vi "Timestamp from dat file.vi"(10 "dat file path":path) -> (2 "time stamp":timestamp)   [LabVIEW 2018]
uses:
  <vilib>/Utility/miscctls.llb/LVDateTimeRec.ctl
panel:
  in  "date time rec":T1
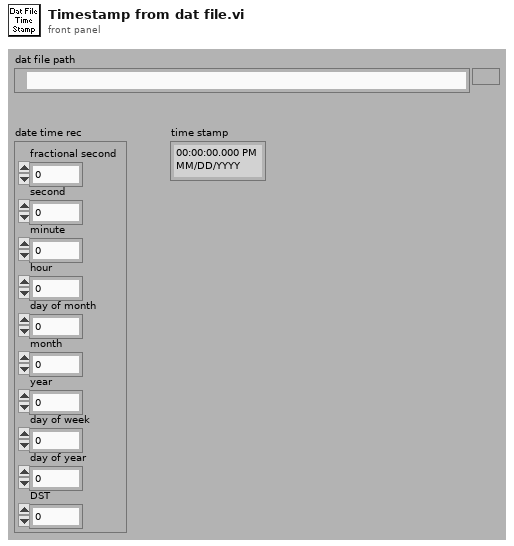
[diagram p1: front panel]
types:
  T1 = typedef "LVDateTimeRec.ctl" = cluster{"fractional second":dbl, "second":i32, "minute":i32, "hour":i32, "day of month":i32, "month":i32, "year":i32, "day of week":i32, "day of year":i32, "DST":i32}
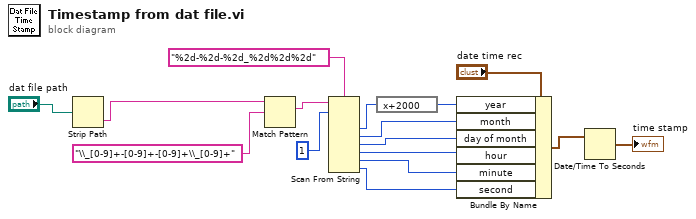
[diagram p0: block diagram]
diagram:
  n1 = Strip Path(path="dat file path") -> (name=w5:string)  [unwired: 1 out]
  n2 = Match Pattern(string=w5, regular expression="\\_[0-9]+-[0-9]+-[0-9]+\\_[0-9]+") -> (match substring=w2:string)  [unwired: 1 in, 3 out]
  n3 = Scan From String(format string="%2d-%2d-%2d_%2d%2d%2d", input string=w2, initial scan location=u32 1) -> (output 1=w15:i32, output 2=w13:i32, output 3=w12:i32, output 4=w11:i32, output 5=w10:i32, output 6=w9:i32)  [unwired: 7 in, 3 out]
  n4 = expression code="x+2000"(w15) -> (w14:i32)
  n5 = Bundle By Name(cluster="date time rec", "year"=w14, "month"=w13, "day of month"=w12, "hour"=w11, "minute"=w10, "second"=w9) -> (w8:T1)
  n6 = Date/Time To Seconds(2:w8) -> (0:→"time stamp":timestamp)  [unwired: 1 in]
